vi "Out_S2F17.vi"(8 "error in (no error)":errorcluster, 11 "S2 Message Class in":refnum<class "S2 Message Class.lvclass">) -> (0 "error out":errorcluster, 3 "S2 Message Class out":refnum<class "S2 Message Class.lvclass">)   [LabVIEW 2020, in "SECS Communication.lvlib" / "S2 Message Class.lvclass"]
uses:
  S2 Message Class.lvclass
  D:/Dropbox/SECS/SECS_GEM v1.0.6/Com/SECS Communication/SECS-II Class/SECS-II Class.lvclass
  SECS-II Class/SECS-II Class.lvclass
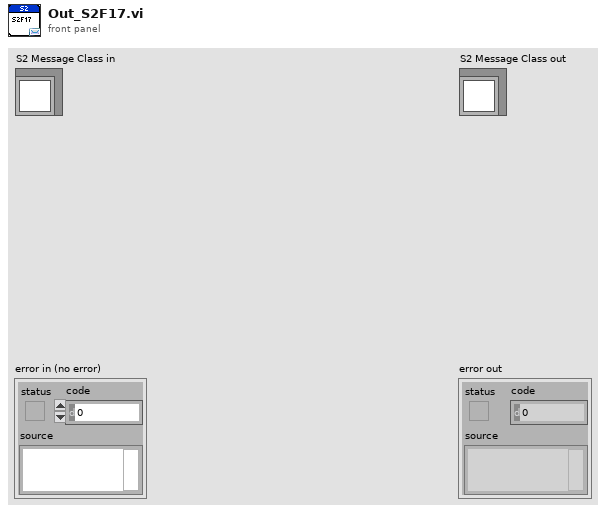
[diagram p1: front panel]
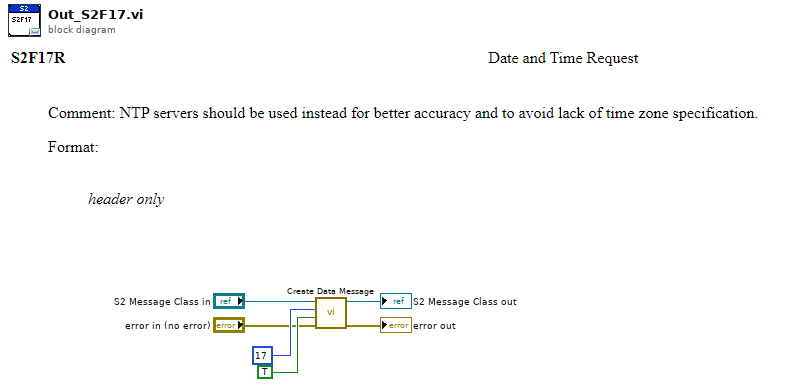
[diagram p0: block diagram]
diagram:
  n1 = call "Create Data Message.vi"("error in (no error)"="error in (no error)", "W-Bit"=TRUE, "Function"=u8 17, "SECS-II Class in"="S2 Message Class in") -> ("error out"=→"error out":errorcluster, "SECS-II Class out"=→"S2 Message Class out":refnum<class "S2 Message Class.lvclass">)  [unwired: 6 in]
